vi "GetSRdata.vi"(8 "Error In":errorcluster, 11 "DBref":T1) -> (0 "Error Out":errorcluster, 2 "SRList":T2 {"SR#" format="%#_10g"})   [LabVIEW 2017, in "Server.lvlib" / "Oracle.lvlib"]
uses:
  Oracle.lvlib
  TypeDefs/SR List.ctl
  TypeDefs/SR Data.ctl
  <vilib>/addons/database/Connection.llb/Conn ObjectReference.ctl
  <vilib>/addons/database/Connection.llb/Conn Execute.vi
  <vilib>/addons/database/Recordset.llb/Rec Fetch Recordset Data (R).vi
  <vilib>/addons/database/Recordset.llb/Rec Destroy - Connection.vi
  <vilib>/addons/database/NI_Database_API.lvlib
  Server.lvlib
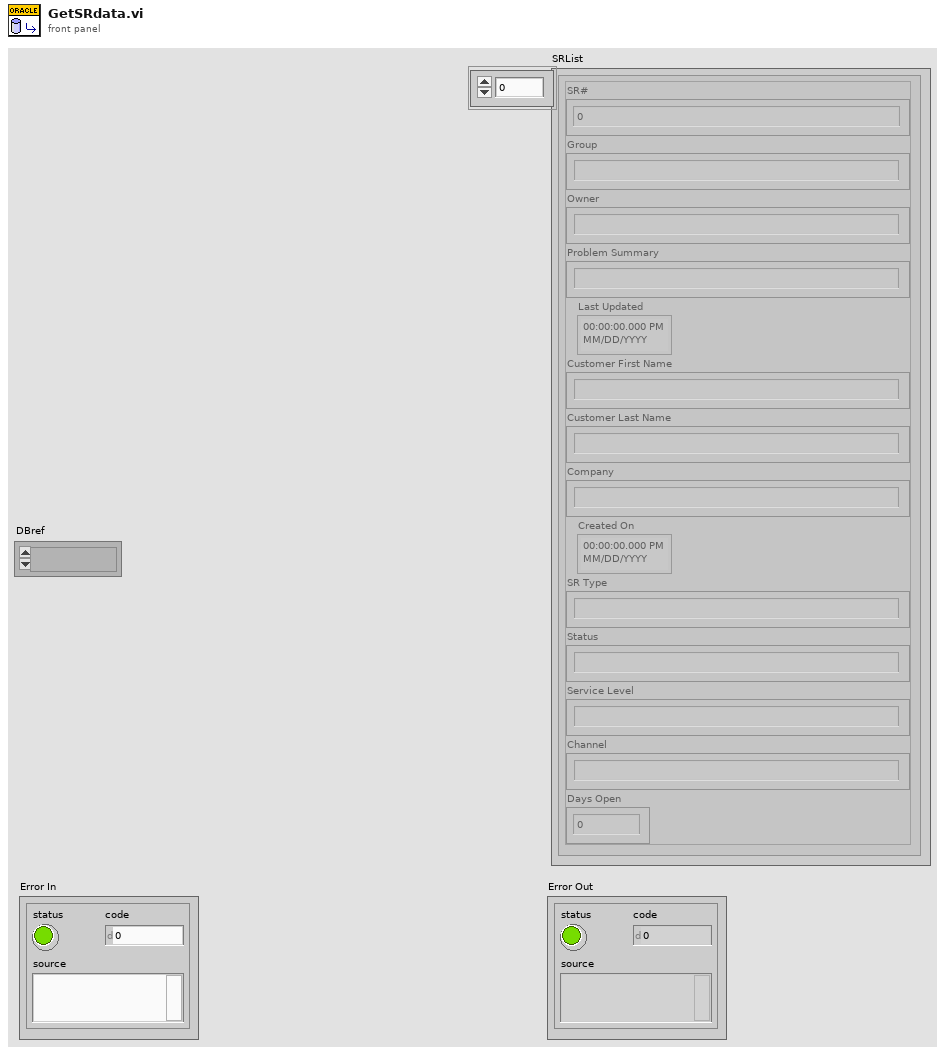
[diagram p1: front panel]
types:
  T1 = typedef "NI_Database_API.lvlib/Conn ObjectReference.ctl" = refnum<k1>
  T2 = typedef "Server.lvlib/SR List.ctl" = T3[]
  T3 = typedef "Server.lvlib/SR Data.ctl" = cluster{"SR#":dbl, "Group":string, "Owner":string, "Problem Summary":string, "Last Updated":timestamp, "Customer First Name":string, "Customer Last Name":string, "Company":string, "Created On":timestamp, "SR Type":string, "Status":string, "Service Level":string, "Channel":string, "Days Open":dbl}
  T4 = typedef "NI_Database_API.lvlib/Rec ObjectReference.ctl" = refnum<k1>
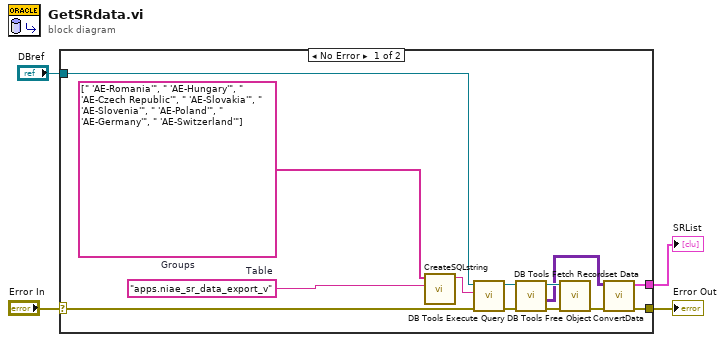
[diagram p0: block diagram]
diagram:
  n1 = case shown="No Error" "Error In" {
    selector: "Error In" -> [w17 w18]
    tunnel: [w6 w18] -> w3
    tunnel: [w11 _] -> w2
    tunnel: "DBref" -> [w12 _]
    frame No Error {
      w5 = "apps.niae_sr_data_export_v"  # Table
      w9 = string[] [" 'AE-Romania'", " 'AE-Hungary'", " 'AE-Czech Republic'", " 'AE-Slovakia'", " 'AE-Slovenia'", " 'AE-Poland'", " 'AE-Germany'", " 'AE-Switzerland'"]  # Groups
      n2 = call "CreateSQLstring.vi"("Table"=w5, "Groups"=w9) -> ("SQL String"=w8:string)  [unwired: 9 in]
      n3 = call-poly <vilib>:"DB Tools Execute Query.vi"("error in (no error)"=w17, "SQL query"=w8, "connection reference"=w12) -> ("error out"=w16:errorcluster, "recordset reference"=w13:T4)  [unwired: 5 in]
      n4 = call-poly <vilib>:"DB Tools Fetch Recordset Data.vi"("error in (no error)"=w16, "recordset reference"=w13) -> ("error out"=w15:errorcluster, "recordset data"=w10:variant[][], "recordset reference out"=w14:T4)  [unwired: 3 in]
      n5 = call-poly <vilib>:"DB Tools Free Object.vi"("error in (no error)"=w15, "recordset reference"=w14) -> ("error out"=w7:errorcluster)  [unwired: 8 in, 1 out]
      n6 = call "ConvertData.vi"("error in (no error)"=w7, "recordset data"=w10) -> ("error out"=w6:errorcluster, "SR List"=w11:T3[])  [unwired: 8 in]
    }
    frame Error {
    }
  }
  "Error Out" <- w3
  "SRList" <- w2
